vi "OpenScope.vi"(0 "Acquisition Unit in (0)":i32, 5 "Acquire Defn In":T1={"Acquire Mode"=enum."stop", "Acquisition mode"=enum."Sampled", "Acquirer"=enum."Cleverscope", "Transfer Chans"=enum."Chan A+B", "A max scale"=5.0, "A min scale"=-5.0, "B max scale"=5.0, "B min scale"=-5.0, "A Probe"=enum."x1", "B Probe"=enum."x1", "A Coupling"=enum."DC", "B Coupling"=enum."DC", "A Bandwidth"=1, "B Bandwidth"=1, "Trigger Source"=enum."Chan A", "Trigger Amplitude"=0.0, "A Trigger Amplitude"=0.0, "B Trigger Amplitude"=0.0, "Trigger Filter"=enum."None", "Trig Slope"=FALSE, "Trigger Holdoff"=0.0, "Dig Pattern Rqd"=FALSE, "Dig Pattern"=0, "Ext Trig Threshold"=0.0, "Dig Input Threshold"=0.0, "Start Time"=-0.003, "Stop Time"=0.003, "Pre Trig Time"=0.003, "Port"=enum."Port 1", "Num divisions"=6, "Num seq frames"=1, "Num Buffers"=2, "Sig Gen Freq"=1000.0, "Sig Gen Amp"=1.0, "Sig Gen Offset"=0.0, "Sig Gen Waveform"=enum."sine", "Sig Gen Sweep"=enum."Log", "Sig Gen Func"=enum."Standard", "Sig Gen Freq 2"=1000.0, "Sig Gen Phase"=180.0, "Trig 2 Function"=enum."None", "Min Trigger Period"=1e-08, "Max trigger Period"=0.0001, "Trigger count"=1, "Trig 2 Slope"=FALSE, "Trig 2 Source Chan"=enum."Chan A", "Trig 2 Level"=0.0, "Dig Pattern 2 Rqd"=FALSE, "Dig Pattern 2"=0, "Trigger 2 Source"=enum."Trigger 1 inverted", "Waveform Averages"=0, "Value changed"=0, "Freq Span"=0.0, "Freq Res"=0.0, "Duration"=0.0, "Resolution"=0.0, "Link Port"=enum."Debug", "Ext Sample Clock"=FALSE, "F Spare 2"=FALSE, "F Spare 3"=FALSE, "F Spare 4"=FALSE, "Sampler Resolution"=enum."10 bit", "Intf Source"=enum."USB", "Update Rate"=enum."20 Frame/sec", "Transfer Size"=enum."Normal", "Sig Gen Freq Step"=0.0, "TCP Adr"=0, "TCP port"=0, "CAU Ser Num Hi"=0, "CAU Ser Num Lo"=0, "Function Number"=0.0, "Function Parameter"=0.0, "Function Result"=0.0, "Link Start"=0, "Link Timebase"=0, "Link Timer"=0, "Link Setup"=0, "Spare 1"=0.0, "Spare 2"=0.0, "Spare 3"=0.0, "Spare 4"=0.0} {"Function Result" format="%#.6p"; "Function Parameter" format="%#.6p"; "Function Number" format="%#.6p"; "TCP Adr" format="%08x"; "Sig Gen Freq Step" format="%.2f"; "Sig Gen Phase" format="%.2f"; "Sig Gen Freq 2" format="%.2f"; "Resolution" format="%#.6p"; "Duration" format="%#.6p"; "Freq Res" format="%#.6p"; "Freq Span" format="%#.6p"; "Dig Pattern 2" format="%.0x"; "Trig 2 Level" step=0.001 format="%#.6p"; "Trigger count" step=1; "Max trigger Period" min=1e-08 max=42.9 step=0.01 format="%#.6p"; "Min Trigger Period" min=1e-08 max=42.9 step=0.01 format="%#_6p"; "Sig Gen Offset" format="%.2f"; "Sig Gen Amp" format="%.2f"; "Sig Gen Freq" format="%.2f"; "B Trigger Amplitude" format="%.1p"; "A Trigger Amplitude" format="%.1p"; "B Bandwidth" format="%x"; "A Bandwidth" format="%x"; "B min scale" format="%.2p"; "B max scale" format="%.2p"; "A min scale" format="%.2p"; "A max scale" format="%.2p"; "Trigger Holdoff" format="%.1p"; "Dig Input Threshold" format="%.2f"; "Ext Trig Threshold" format="%.2f"; "Dig Pattern" format="%.0x"; "Pre Trig Time" format="%.3p"; "Start Time" format="%.2p"; "Trigger Amplitude" format="%.1p"; "Stop Time" format="%.2p"}, 11 "error in":errorcluster) -> (4 "Acquisition Unit out":i32, 6 "Acquire Defn Out":T1={"Acquire Mode"=enum."stop", "Acquisition mode"=enum."Sampled", "Acquirer"=enum."Cleverscope", "Transfer Chans"=enum."Chan A+B", "A max scale"=5.0, "A min scale"=-5.0, "B max scale"=5.0, "B min scale"=-5.0, "A Probe"=enum."x1", "B Probe"=enum."x1", "A Coupling"=enum."DC", "B Coupling"=enum."DC", "A Bandwidth"=1, "B Bandwidth"=1, "Trigger Source"=enum."Chan A", "Trigger Amplitude"=0.0, "A Trigger Amplitude"=0.0, "B Trigger Amplitude"=0.0, "Trigger Filter"=enum."None", "Trig Slope"=FALSE, "Trigger Holdoff"=0.0, "Dig Pattern Rqd"=FALSE, "Dig Pattern"=0, "Ext Trig Threshold"=0.0, "Dig Input Threshold"=0.0, "Start Time"=-0.003, "Stop Time"=0.003, "Pre Trig Time"=0.003, "Port"=enum."Port 1", "Num divisions"=6, "Num seq frames"=1, "Num Buffers"=2, "Sig Gen Freq"=1000.0, "Sig Gen Amp"=1.0, "Sig Gen Offset"=0.0, "Sig Gen Waveform"=enum."sine", "Sig Gen Sweep"=enum."Linear", "Sig Gen Func"=enum."Standard", "Sig Gen Freq 2"=1000.0, "Sig Gen Phase"=180.0, "Trig 2 Function"=enum."None", "Min Trigger Period"=1e-08, "Max trigger Period"=0.0001, "Trigger count"=1, "Trig 2 Slope"=FALSE, "Trig 2 Source Chan"=enum."Chan A", "Trig 2 Level"=0.0, "Dig Pattern 2 Rqd"=FALSE, "Dig Pattern 2"=0, "Trigger 2 Source"=enum."Trigger 1 inverted", "Waveform Averages"=0, "Value changed"=0, "Freq Span"=0.0, "Freq Res"=0.0, "Duration"=0.0, "Resolution"=0.0, "Link Port"=enum."Debug", "Ext Sample Clock"=FALSE, "F Spare 2"=FALSE, "F Spare 3"=FALSE, "F Spare 4"=FALSE, "Sampler Resolution"=enum."10 bit", "Intf Source"=enum."USB", "Update Rate"=enum."20 Frame/sec", "Transfer Size"=enum."Normal", "Sig Gen Freq Step"=10.0, "TCP Adr"=0, "TCP port"=0, "CAU Ser Num Hi"=0, "CAU Ser Num Lo"=0, "Function Number"=0.0, "Function Parameter"=0.0, "Function Result"=0.0, "Link Start"=0, "Link Timebase"=0, "Link Timer"=0, "Link Setup"=0, "Spare 1"=0.0, "Spare 2"=0.0, "Spare 3"=0.0, "Spare 4"=0.0} {"Function Result" format="%#.6p"; "Function Parameter" format="%#.6p"; "Function Number" format="%#.6p"; "TCP Adr" format="%08x"; "Sig Gen Freq Step" format="%.2f"; "Sig Gen Phase" format="%.2f"; "Sig Gen Freq 2" format="%.2f"; "Resolution" format="%#.6p"; "Duration" format="%#.6p"; "Freq Res" format="%#.6p"; "Freq Span" format="%#.6p"; "Dig Pattern 2" format="%.0x"; "Trig 2 Level" step=0.001 format="%#.6p"; "Trigger count" step=1; "Max trigger Period" min=1e-08 max=42.9 step=0.01 format="%#.6p"; "Min Trigger Period" min=1e-08 max=42.9 step=0.01 format="%#_6p"; "Sig Gen Offset" format="%.2f"; "Sig Gen Amp" format="%.2f"; "Sig Gen Freq" format="%.2f"; "B Trigger Amplitude" format="%.1p"; "A Trigger Amplitude" format="%.1p"; "B Bandwidth" format="%x"; "A Bandwidth" format="%x"; "B min scale" format="%.2p"; "B max scale" format="%.2p"; "A min scale" format="%.2p"; "A max scale" format="%.2p"; "Trigger Holdoff" format="%.1p"; "Dig Input Threshold" format="%.2f"; "Ext Trig Threshold" format="%.2f"; "Dig Pattern" format="%.0x"; "Pre Trig Time" format="%.3p"; "Start Time" format="%.2p"; "Trigger Amplitude" format="%.1p"; "Stop Time" format="%.2p"}, 14 "CAU status":T17, 15 "error out":errorcluster)   [LabVIEW 2009]
uses:
  libraries/Cscope control driver.llb/Cscope intf status.ctl
  libraries/Cscope control driver.llb/Acquire Event type.ctl
  libraries/Cscope control driver.llb/Acquire capture type.ctl
  libraries/Cscope control driver.llb/Acquire capture method.ctl
  libraries/Cscope control driver.llb/Acquirer type.ctl
  libraries/Cscope control driver.llb/Input Range.ctl
  libraries/Cscope control driver.llb/Input Coupling.ctl
  libraries/Cscope control driver.llb/Input Bandwidth.ctl
  libraries/Cscope control driver.llb/USB channel.ctl
  libraries/Cscope control driver.llb/Trigger Filter.ctl
  libraries/Cscope control driver.llb/Cscope waveform type.ctl
  libraries/Cscope control driver.llb/Trigger Period.ctl
  libraries/Cscope control driver.llb/Trigger channel.ctl
  libraries/Cscope control driver.llb/Link port types.ctl
  libraries/Cscope control driver.llb/Acquirer resolution.ctl
  libraries/Cscope control driver.llb/Intf source.ctl
  libraries/Cscope control driver.llb/Acquire transfer size.ctl
  libraries/Cscope control driver.llb/Cscope control command type.ctl
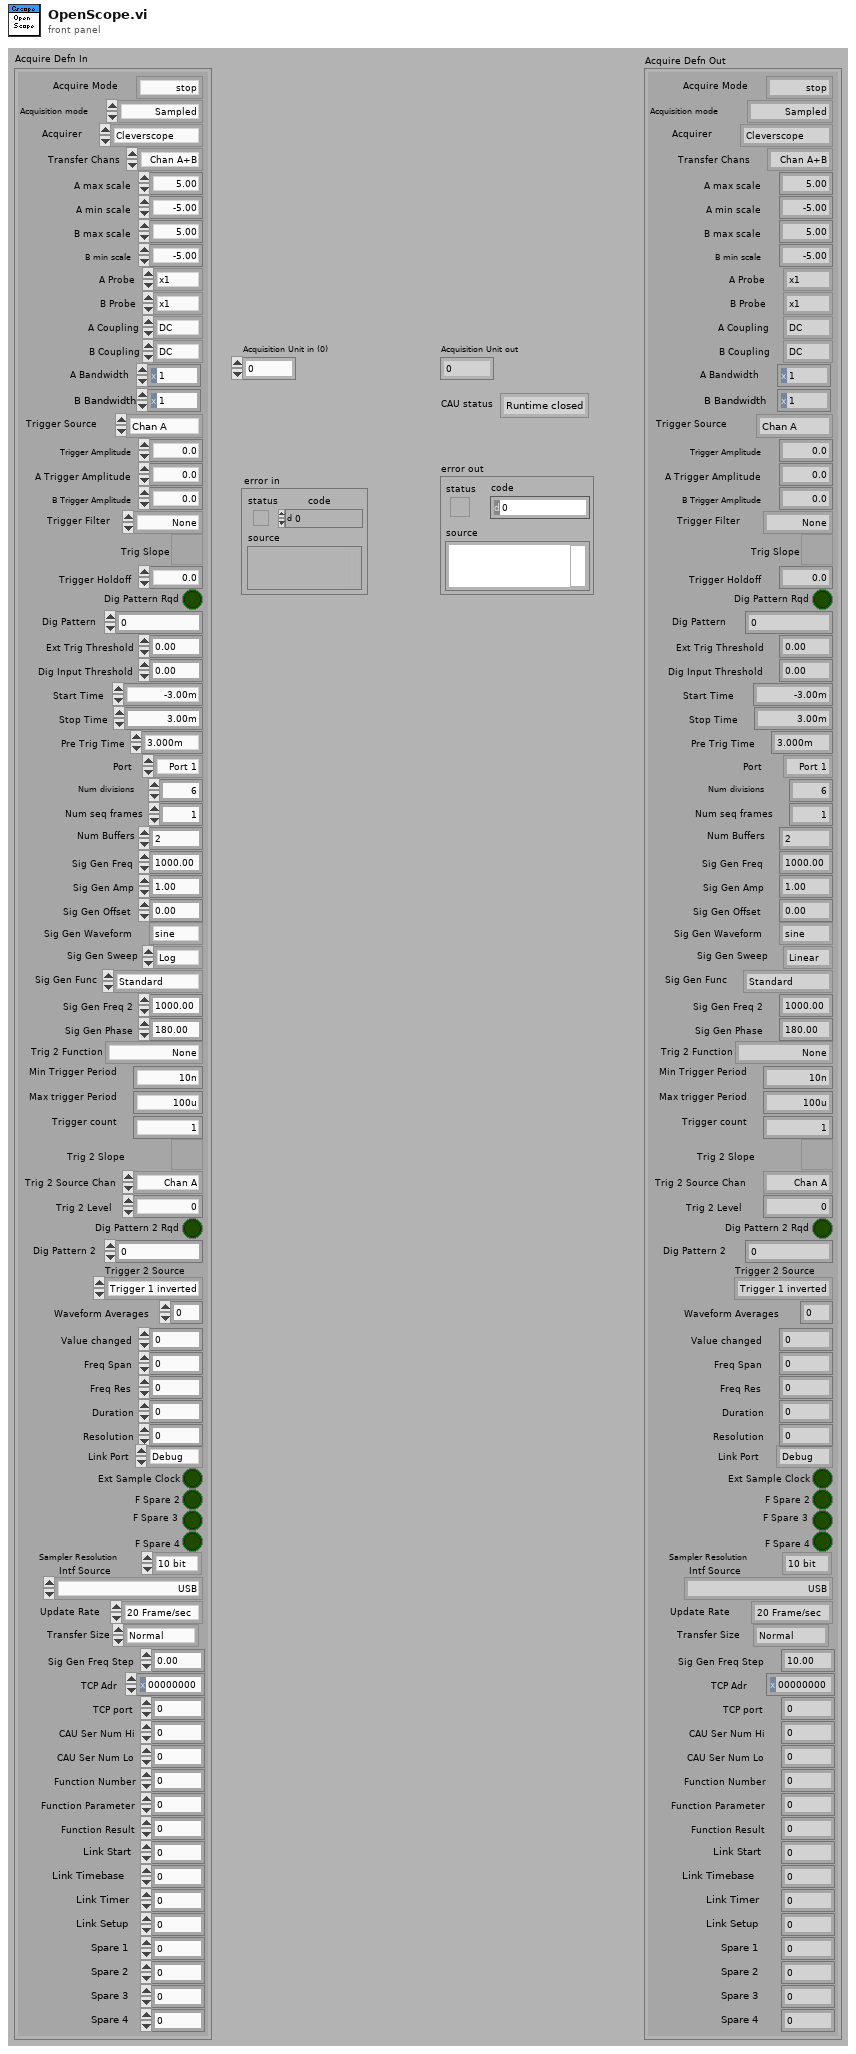
[diagram p1: front panel]
types:
  T1 = typedef "Acquire Event type.ctl" = cluster{"Acquire Mode":T2, "Acquisition mode":T3, "Acquirer":T4, "Transfer Chans":enum16{"Chan A", "Chan B", "Chan A+B"}, "A max scale":dbl, "A min scale":dbl, "B max scale":dbl, "B min scale":dbl, "A Probe":T5, "B Probe":T5, "A Coupling":T6, "B Coupling":T6, "A Bandwidth":T7, "B Bandwidth":T7, "Trigger Source":T8, "Trigger Amplitude":dbl, "A Trigger Amplitude":dbl, "B Trigger Amplitude":dbl, "Trigger Filter":T9, "Trig Slope":bool, "Trigger Holdoff":dbl, "Dig Pattern Rqd":bool, "Dig Pattern":u32, "Ext Trig Threshold":dbl, "Dig Input Threshold":dbl, "Start Time":dbl, "Stop Time":dbl, "Pre Trig Time":dbl, "Port":enum16{"Port 1", "Port 2", "Port 3", "Port 4", "Port 5", "Port 6"}, "Num divisions":i16, "Num seq frames":i16, "Num Buffers":i32, "Sig Gen Freq":dbl, "Sig Gen Amp":dbl, "Sig Gen Offset":dbl, "Sig Gen Waveform":T10, "Sig Gen Sweep":enum16{"Linear", "Log"}, "Sig Gen Func":enum16{"Standard", "Auto advance", "Freq mod In8", "Phase mod In8"}, "Sig Gen Freq 2":dbl, "Sig Gen Phase":dbl, "Trig 2 Function":T11, "Min Trigger Period":dbl, "Max trigger Period":dbl, "Trigger count":u32, "Trig 2 Slope":bool, "Trig 2 Source Chan":T12, "Trig 2 Level":dbl, "Dig Pattern 2 Rqd":bool, "Dig Pattern 2":u32, "Trigger 2 Source":enum16{"Trigger 1 inverted", "Trig 2 Defn"}, "Waveform Averages":i32, "Value changed":i32, "Freq Span":dbl, "Freq Res":dbl, "Duration":dbl, "Resolution":dbl, "Link Port":T13, "Ext Sample Clock":bool, "F Spare 2":bool, "F Spare 3":bool, "F Spare 4":bool, "Sampler Resolution":T14, "Intf Source":T15, "Update Rate":enum16{"20 Frame/sec", "10 Frame/sec", "5 Frame/sec"}, "Transfer Size":T16, "Sig Gen Freq Step":dbl, "TCP Adr":u32, "TCP port":u32, "CAU Ser Num Hi":u32, "CAU Ser Num Lo":u32, "Function Number":dbl, "Function Parameter":dbl, "Function Result":dbl, "Link Start":u32, "Link Timebase":u32, "Link Timer":u32, "Link Setup":u32, "Spare 1":dbl, "Spare 2":dbl, "Spare 3":dbl, "Spare 4":dbl}
  T2 = typedef "Acquire capture type.ctl" = enum16{"single", "automatic", "triggered", "stop", "single stop", "replay"}
  T3 = typedef "Acquire capture method.ctl" = enum16{"Sampled", "Peak Captured", "Filtered", "Repetitive", "Waveform avg"}
  T4 = typedef "Acquirer type.ctl" = enum16{"Internal Sig Gen", "APC 901", "APC 901A", "Sound Card", "Cleverscope"}
  T5 = typedef "Input Range.ctl" = enum16{"x1", "x10", "x100", "x1K", "x20", "x50", "x200"}
  T6 = typedef "Input Coupling.ctl" = enum16{"AC", "DC"}
  T7 = typedef "Input Bandwidth.ctl" = u16
  T8 = typedef "USB channel.ctl" = enum32{"Chan A", "Chan B", "Ext Trigger", "Dig Trig", "Link Input", "chan_5", "chan_6", "chan_7", "chan_8", "chan_9", "chan_10", "chan_11", "chan_12", "chan_13", "chan_14", "chan_15"}
  T9 = typedef "Trigger Filter.ctl" = enum16{"None", "Low Pass", "Hi Pass", "Noise"}
  T10 = typedef "Cscope waveform type.ctl" = enum16{"sine", "triangle", "square", "DC", "OFF"}
  T11 = typedef "Trigger Period.ctl" = enum16{"None", "Trig 1~2 < min", "min<T1~2 < max", "Trig 1~2 > max", "Count Trig 1", "Count Trig 2"}
  T12 = typedef "Trigger channel.ctl" = enum32{"Chan A", "Chan B", "Ext Trigger", "Dig Trig", "Link Input"}
  T13 = typedef "Link port types.ctl" = enum8{"Debug", "Link Out", "Disabled", "Slave", "Master", "Uart", "SPI", "I2C", "Digital", "Sig Gen"}
  T14 = typedef "Acquirer resolution.ctl" = enum16{"10 bit", "12 Bit", "14 bit"}
  T15 = typedef "Intf source.ctl" = enum16{"USB", "Ethernet - Find by IP address", "Ethernet - Find first IP address", "Ethernet - Find by serial number"}
  T16 = typedef "Acquire transfer size.ctl" = enum16{"Normal", "100% Buffer", "50% Buffer", "10% Buffer", "5% Buffer", "2% Buffer", "Sequence"}
  T17 = typedef "Cscope intf status.ctl" = enum16{"Runtime closed", "Closed", "Open", "Fault", "Fault closed"}
  T18 = typedef "Cscope control command type.ctl" = enum16{"Initialize", "Acquire", "Replay", "Wait for samples", "Update", "Close", "Status", "Function", "Get Frame", "Finish", "Function Result", "Check Got Samples", "Get Chan A", "Get Chan B", "Get Dig"}
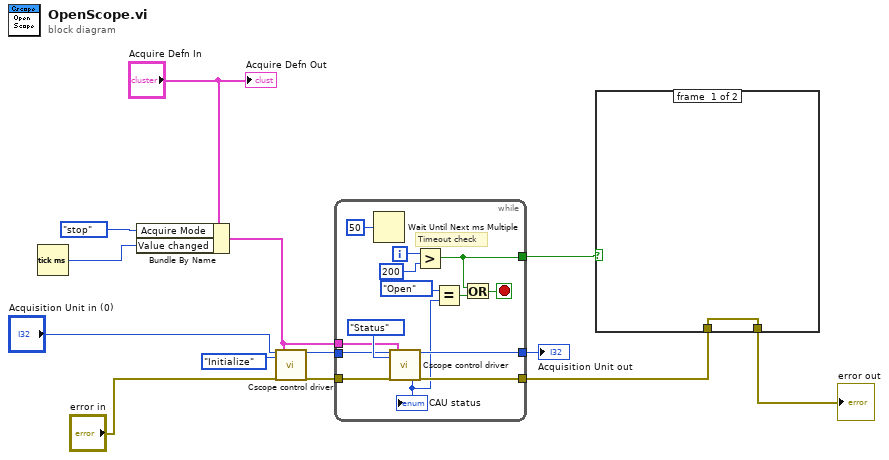
[diagram p0: block diagram]
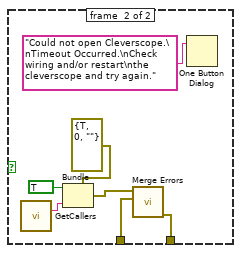
[diagram p2: hidden frame]
diagram:
  n1 = Tick Count (ms)() -> (millisecond timer value=w6:u32)
  n2 = Bundle By Name(cluster="Acquire Defn In", "Acquire Mode"=Acquire_capture_type."stop", "Value changed"=w6) -> (w5:T1)
  n3 = call "Cscope control driver.vi"("Acquisition Unit in"="Acquisition Unit in (0)", "Command"=Cscope_control_command_type."Initialize", "error in"="error in", "Acquire Definition"=w5) -> ("Acquisition Unit out"=w10:i32, "error out"=w12:errorcluster)  [unwired: 4 in, 10 out]
  n4 = while {
    tunnel: w12 -> [w27]
    tunnel: [w26] -> w2
    tunnel: [w17] -> w9
    tunnel: w10 -> [w18]
    tunnel: w5 -> [w15]
    tunnel: [w14] -> w4
    i -> [w24]
    stop <- w21 stop-if-true
    # "Timeout check"
    n5 = Wait Until Next ms Multiple(millisecond multiple=u32 50) -> ()  [unwired: 1 out]
    n6 = call "Cscope control driver.vi"("Acquisition Unit in"=w18, "Command"=Cscope_control_command_type."Status", "error in"=w27, "Acquire Definition"=w15) -> ("CAU status"=w16:T17, "Acquisition Unit out"=w17:i32, "error out"=w26:errorcluster)  [unwired: 4 in, 9 out]
    "CAU status" <- w16
    n7 = Greater?(x=w24, y=200) -> (0:w14:bool)
    n8 = Equal?(x=Cscope_intf_status."Open", y=w16) -> (x = y?=w20:bool)
    n9 = Or(x=w14, y=w20) -> (x .or. y?=w21:bool)
  }
  "Acquisition Unit out" <- w9
  n10 = case shown="True" w4 {
    tunnel: w2 -> [w28 w34]
    tunnel: [w28 w35] -> w1
    frame #0 {
    }
    frame #1 {
      n11 = call "GetCallers.vi"() -> ("Caller String"=w29:string)  [unwired: 15 in]
      n12 = Bundle(cluster=errorcluster {"status"=TRUE, "code"=0, "source"=""} ("error out"), "status"=TRUE, "source"=w29) -> (w32:errorcluster)  [unwired: 1 in]
      n13 = call <vilib>:"Merge Errors.vi"("error in 2 (no error)"=w34, "error in 1 (no error)"=w32) -> ("error out"=w35:errorcluster)  [unwired: 5 in]
      n14 = One Button Dialog(message="Could not open Cleverscope.\nTimeout Occurred.\nCheck wiring and/or restart\nthe cleverscope and try again.") -> ()  [unwired: 1 in, 1 out]
    }
  }
  "error out" <- w1
  "Acquire Defn Out" <- "Acquire Defn In"
